vi "PositMeanDist.vi"(8 "Count":i32=3, 11 "Posit Array":T1[](array[typedef])) -> (0 "Array size":i32, 1 "mean":dbl format="%0.2f", 2 "Latest dist":dbl format="%0.2f", 3 "Posit Array":T1[](array[typedef]))   [LabVIEW 2014]
uses:
  Libraries/Contact Data/Position.ctl
  <vilib>/Analysis/baseanly.llb/Mean (DBL).vi
  <vilib>/Analysis/NI_AALBase.lvlib
  Libraries/Contact Data/Contact Data.lvlib
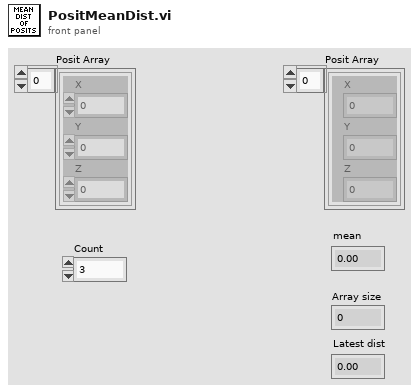
[diagram p1: front panel]
types:
  T1 = typedef "Contact Data.lvlib/Position.ctl" = cluster{"X":dbl, "Y":dbl, "Z":dbl}
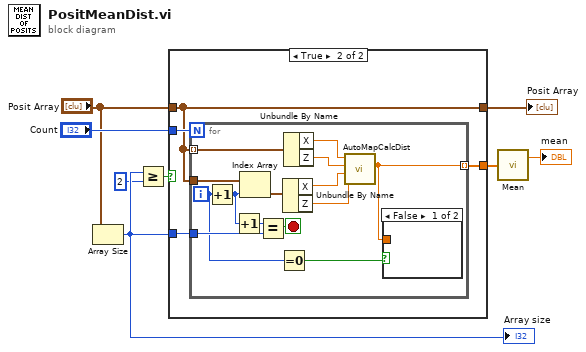
[diagram p0: block diagram]
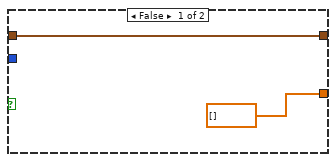
[diagram p2: hidden frame]
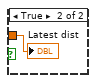
[diagram p3: hidden frame]
diagram:
  n1 = Array Size(array="Posit Array") -> (size(s)=w5:i32)
  "Array size" <- w5
  n2 = Greater Or Equal?(x=w5, y=2) -> (x >= y?=w3:bool)
  n3 = case shown="True" w3 {
    tunnel: "Posit Array" -> [w10 w11]
    tunnel: w5 -> [_ w14]
    tunnel: [dbl[] [] w13] -> w8
    tunnel: [w10 w11] -> w6
    tunnel: "Count" -> [_ w12]
    frame False {
    }
    frame True {
      n4 = for {
        N: w12 -> [_]
        tunnel: w11 -> [w28] mode=indexing
        tunnel: w11 -> [w27]
        tunnel: w14 -> [w20]
        tunnel: [w15] -> w13 mode=indexing
        i -> [w17]
        stop <- w19 stop-if-true
        n5 = Increment(x=w17) -> (x+1=w21:i32)
        n6 = Increment(x=w21) -> (x+1=w18:i32)
        n7 = Index Array(array=w27, index=w21) -> (element=w26:T1)
        n8 = Equal?(x=w18, y=w20) -> (x = y?=w19:bool)
        n9 = Equal To 0?(x=w17) -> (x = 0?=w16:bool)
        n10 = Unbundle By Name(w26) -> ("X"=w23:dbl, "Z"=w22:dbl)
        n11 = Unbundle By Name(w28) -> ("X"=w25:dbl, "Z"=w24:dbl)
        n12 = call "AutoMapCalcDist.vi"("Y2"=w22, "X2"=w23, "Y1"=w24, "X1"=w25) -> ("Distance"=w15:dbl)  [unwired: 7 in]
        n13 = case shown="False" w16 {
          tunnel: w15 -> [_ w29]
          frame False {
          }
          frame True {
            "Latest dist" <- w29
          }
        }
      }
    }
  }
  "Posit Array" <- w6
  n14 = call-poly <vilib>:"Mean.vi"("X"=w8) -> ("mean"=→"mean":dbl)  [unwired: 1 out]
